vi "Batch Convert RGB565.vi"(8 "error in":errorcluster, 10 "folder to output file":path=path "D:/CASE/Mars Rover/Working Directory/osr-rover-code/OsrScreen/emoji_16x32_source", 11 "folder to image files (png, jpeg, jpg, bmp)":path=path "D:/CASE/Mars Rover/Working Directory/osr-rover-code/OsrScreen/Osr_Screen_Face/Images/emoji_16x32") -> (0 "error out":errorcluster)   [LabVIEW 2019, in "LabVIEW RGB565 Convertor.lvlib"]
uses:
  LabVIEW RGB565 Convertor.lvlib
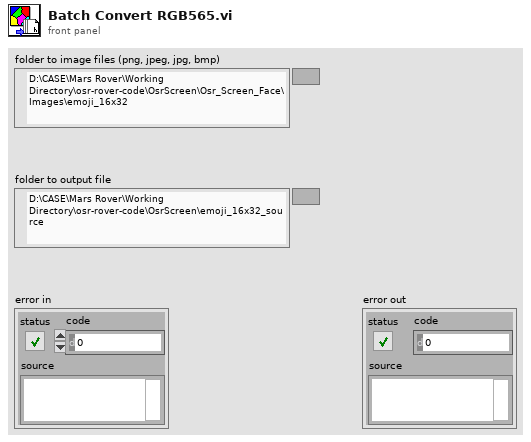
[diagram p1: front panel]
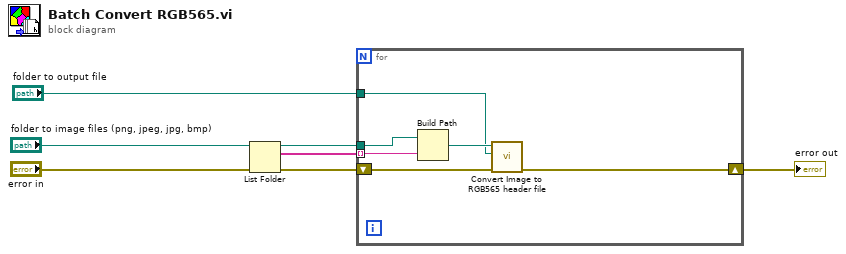
[diagram p0: block diagram]
diagram:
  n1 = List Folder(path="folder to image files (png, jpeg, jpg, bmp)", error in="error in") -> (path out=w4:path, filenames=w5:string[], error out=w3:errorcluster)  [unwired: 2 in, 1 out]
  n2 = for {
    tunnel: w5 -> [w12] mode=indexing
    tunnel: w4 -> [w13]
    tunnel: "folder to output file" -> [w9]
    shift-right: [w8] -> w1
    shift-left: w3 -> [w10]
    n3 = Build Path(base path=w13, name or relative path=w12) -> (appended path=w11:path)
    n4 = call "Convert Image to RGB565 header file.vi"("error in (no error)"=w10, "folder to output file"=w9, "path to image file (png, jpeg, jpg, bmp)"=w11) -> ("error out"=w8:errorcluster)  [unwired: 8 in]
  }
  "error out" <- w1
